vi "Main Worker.vi"(9 "Read Queue Return":refnum<queue>, 10 "Control Queue Return":refnum<queue>, 11 "Network Session Handler in":refnum<class "Network Session Handler.lvclass">) -> ()   [LabVIEW 2019, in "Network Interface.lvlib" / "Network Session Handler.lvclass"]
uses:
  <vilib>/gpm_packages/@cs/Network-Sink/Source/Network Interface/Network Session Handler/Network Session Handler.lvclass
  <vilib>/gpm_packages/@cs/Network-Sink/Source/Network Interface/Message Queue/Message Queue.lvclass
  <vilib>/gpm_packages/@cs/Network-Sink/Source/Network Interface/Network Session Handler/Network Session Handler.lvclass/Network Session Handler.ctl
  <vilib>/gpm_packages/@cs/Network-Sink/Source/Network Interface/Network Session Handler/Session Handler Message Names ENUM.ctl
  <vilib>/gpm_packages/@cs/Network-Sink/Source/Network Interface/Message Queue/Message Queue.lvclass/Message Queue.ctl
  <vilib>/gpm_packages/@cs/Network-Sink/Source/Network Interface/Network Session Handler/Factory Loop Message Names ENUM.ctl
  <vilib>/gpm_packages/@cs/Network-Sink/Source/Network Interface/Connection Handler/Synchronous Write Request.ctl
  <vilib>/gpm_packages/@cs/event-logger/Source/Composed Log/Types/Log Level.ctl
  <vilib>/gpm_packages/@cs/event-logger/Source/Composed Log/LoggerReference/LoggerReference.lvclass/LoggerReference.ctl
  6a8aa042-a92f-476e-a18a-366c18080255.vi
  510cd40e-2ed8-4bdb-87dc-9d54a7f70cf6.vi
  31b7514c-8e2c-4e78-b35a-21c1860db5bd.vi
  c51e2ab3-c1d1-4a5d-a2cc-0a28ab4f9529.vi
  <vilib>/gpm_packages/@cs/Network-Sink/Source/Network Interface/Message Queue/Protected Enqueue.vi
  <vilib>/gpm_packages/@cs/Network-Sink/Source/Network Interface/Message Queue/Dequeue Message.vi
  <vilib>/gpm_packages/@cs/event-logger/Source/Composed Log/LoggerReference/Log.vi
  <vilib>/gpm_packages/@cs/event-logger/Source/Composed Log/LoggerReference/Get Valid Event Time.vi
  <vilib>/gpm_packages/@cs/event-logger/Source/Composed Log/LoggerReference/Remove Stale Logs.vi
  <vilib>/gpm_packages/@cs/Network-Sink/Source/Network Interface/Connection Handler/Connection Handler.lvclass
  <vilib>/gpm_packages/@cs/event-logger/Source/Composed Log/Composed Log.lvlib
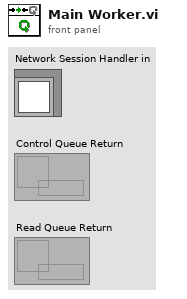
[diagram p1: front panel]
types:
  T1 = typedef "Network Interface.lvlib/Network Session Handler.lvclass/Session Handler Message Names ENUM.ctl" = enum16{"Transmit Message", "Stop", "Handler Shutdown", "Error"}
  T2 = typedef "Network Interface.lvlib/Network Session Handler.lvclass/Factory Loop Message Names ENUM.ctl" = enum16{"Create Connection", "Stop", "Assess Factory State"}
  T3 = typedef "Network Interface.lvlib/Connection Handler.lvclass/Synchronous Write Request.ctl" = cluster{"Data To Write":string, "Return Queue":refnum<queue>}
  T4 = typedef "Composed Log.lvlib/Log Level.ctl" = enum16{"Debug", "Info", "Warning", "Error", "Critical"}
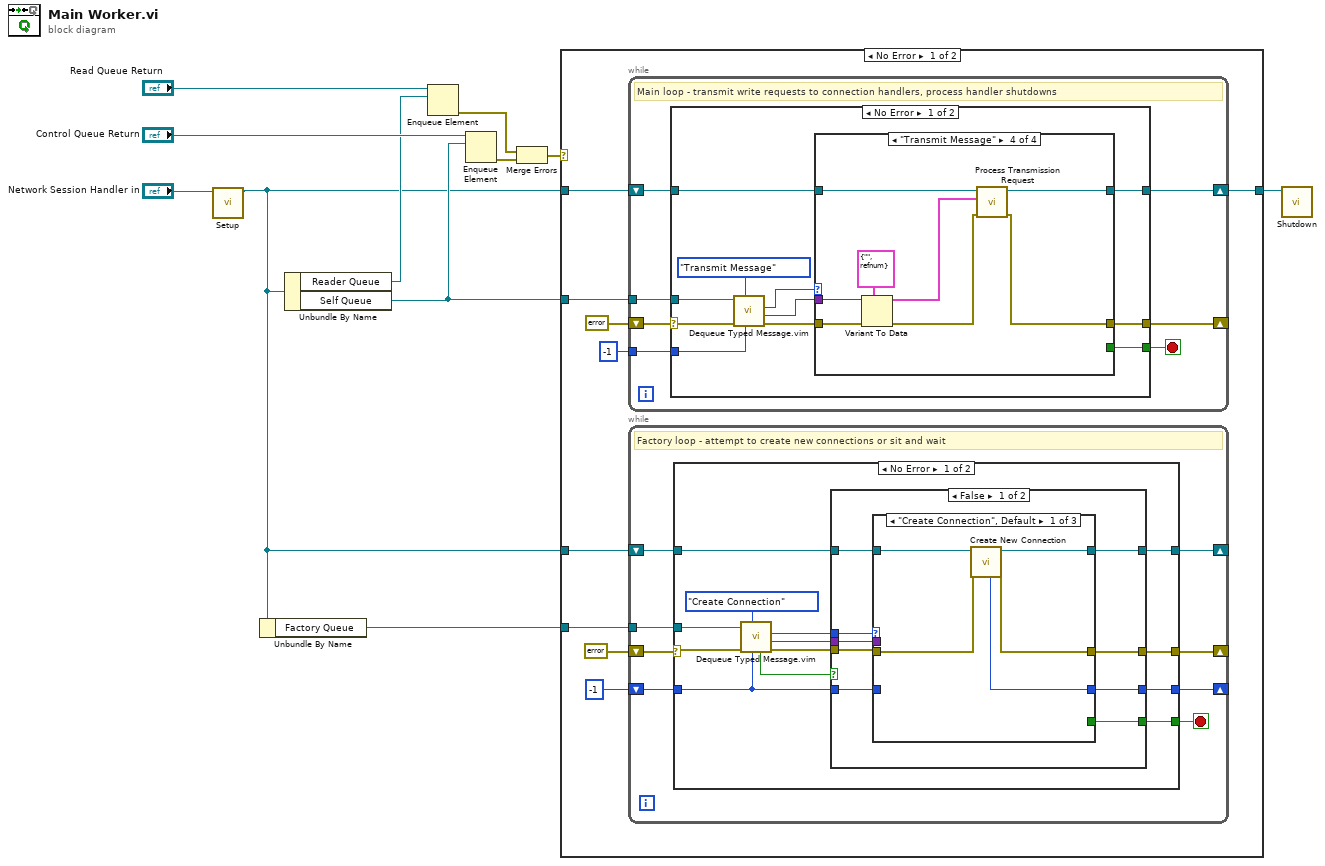
[diagram p0: block diagram]
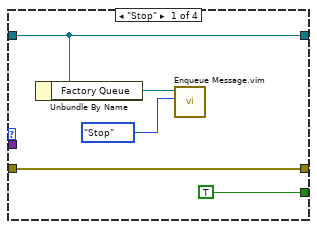
[diagram p2: hidden frame]
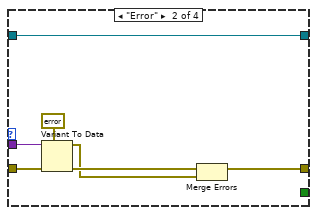
[diagram p3: hidden frame]
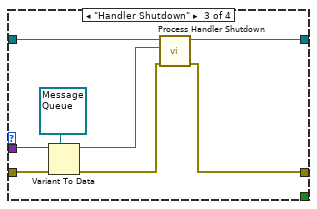
[diagram p4: hidden frame]
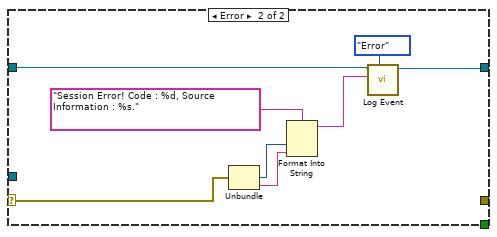
[diagram p5: hidden frame]
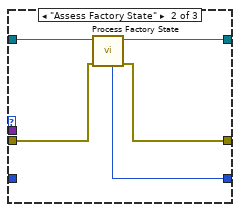
[diagram p6: hidden frame]
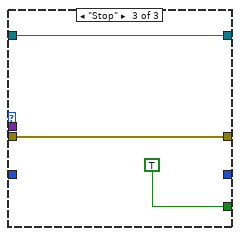
[diagram p7: hidden frame]
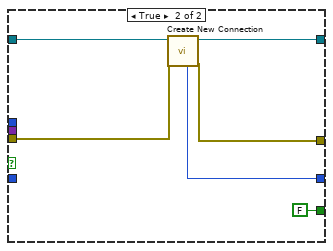
[diagram p8: hidden frame]
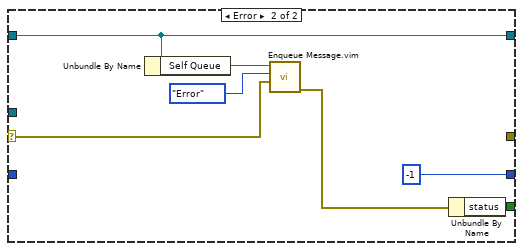
[diagram p9: hidden frame]
diagram:
  n1 = call <vilib>:"Setup.vi"("Network Session Handler in"="Network Session Handler in") -> ("Network Session Handler out"=w1:refnum<class "Network Session Handler.lvclass">)  [unwired: 9 in, 1 out]
  n2 = Unbundle By Name(w1) -> ("Factory Queue"=w11:refnum<class "Message Queue.lvclass">)
  n3 = Unbundle By Name(w1) -> ("Reader Queue"=w6:refnum<queue>, "Self Queue"=w8:refnum<class "Message Queue.lvclass">)
  n4 = Enqueue Element(queue="Read Queue Return", element=w6) -> (error out=w3:errorcluster)  [unwired: 2 in, 2 out]
  n5 = Enqueue Element(queue="Control Queue Return", element=w8) -> (error out=w5:errorcluster)  [unwired: 2 in, 2 out]
  n6 = Merge Errors(w3, w5) -> (w4:errorcluster)
  n7 = case shown="No Error" w4 {
    tunnel: w11 -> [w19 _]
    tunnel: w1 -> [w16 _]
    tunnel: w8 -> [w15 _]
    tunnel: w1 -> [w14 w131]
    tunnel: [w13 w131] -> w2
    frame No Error {
      n8 = while {
        tunnel: w15 -> [w23]
        shift-right: [w27] -> _
        shift-left: errorcluster {"status"=FALSE, "code"=0, "source"=""} ("error out") -> [w24]
        shift-right: [w25] -> w13
        shift-left: w14 -> [w26]
        tunnel: -1 ("Timeout (-1)") -> [w21]
        stop <- w22 stop-if-true
        # "Main loop - transmit write requests to connection handlers, process handler shutdowns"
        n9 = case shown="No Error" w24 {
          selector: w24 -> [w35 w70]
          tunnel: [w38 _] -> w27
          tunnel: w26 -> [w37 w69]
          tunnel: [w36 w68] -> w25
          tunnel: w23 -> [w34 _]
          tunnel: [w29 _] -> w22
          tunnel: w21 -> [w28 _]
          frame No Error {
            n10 = call "Dequeue Typed Message.vim"("Timeout (-1)"=w28, "Type"=Session_Handler_Message_Names_ENUM."Transmit Message", "error in (no error)"=w35, "Message Queue in"=w34) -> ("error out"=w30:errorcluster, "Data"=w31:variant, "Msg"=w32:T1)  [unwired: 3 in, 2 out]
            n11 = case shown="\"Transmit Message\"" w32 {
              tunnel: w31 -> [_ w48 w56 w65]
              tunnel: w30 -> [w43 w50 w58 w66]
              tunnel: [w43 w45 w52 w59] -> w38
              tunnel: w37 -> [w41 w46 w55 w64]
              tunnel: [w41 w46 w54 w63] -> w36
              tunnel: [TRUE _ _ _] -> w29
              frame "Stop" {
                n12 = Unbundle By Name(w41) -> ("Factory Queue"=w40:refnum<class "Message Queue.lvclass">)
                n13 = call "Enqueue Message.vim"("Msg"=Factory_Loop_Message_Names_ENUM."Stop" ("Factory Message Names"), "Message Queue in"=w40) -> ()  [unwired: 8 in, 2 out]
              }
              frame "Error" {
                n14 = Variant To Data(error in=w50, type=errorcluster {"status"=FALSE, "code"=0, "source"=""} ("error out"), Variant=w48) -> (data=w44:errorcluster, error out=w49:errorcluster)
                n15 = Merge Errors(w49, w44) -> (w45:errorcluster)
              }
              frame "Handler Shutdown" {
                n16 = Variant To Data(error in=w58, type=refnum<class "Message Queue.lvclass"> refnum ("Network Sink.lvlib:Message Queue.lvclass"), Variant=w56) -> (data=w51:refnum<class "Message Queue.lvclass">, error out=w53:errorcluster)
                n17 = call <vilib>:"Process Handler Shutdown.vi"("error in (no error)"=w53, "Handler Queue"=w51, "Network Session Handler in"=w55) -> ("error out"=w52:errorcluster, "Network Session Handler out"=w54:refnum<class "Network Session Handler.lvclass">)  [unwired: 7 in]
              }
              frame "Transmit Message" {
                n18 = Variant To Data(error in=w66, type=T3 {"Data To Write"="", "Return Queue"=refnum} ("Write Request"), Variant=w65) -> (data=w61:T3, error out=w60:errorcluster)
                n19 = call <vilib>:"Process Transmission Request.vi"("error in (no error)"=w60, "Write Request"=w61, "Network Session Handler in"=w64) -> ("error out"=w59:errorcluster, "Network Session Handler out"=w63:refnum<class "Network Session Handler.lvclass">)  [unwired: 7 in]
              }
            }
          }
          frame Error {
            n20 = Unbundle(w70) -> ("code"=w73:i32, "source"=w72:string)  [unwired: 1 out]
            n21 = Format Into String(format string="Session Error! Code : %d, Source Information : %s.", w73, w72) -> (resulting string=w67:string)  [unwired: 2 in, 1 out]
            n22 = call <vilib>:"Log Event.vi"("Event Level"=Log_Level."Error", "Event"=w67, "Network Session Handler in"=w69) -> ("Network Session Handler out"=w68:refnum<class "Network Session Handler.lvclass">)  [unwired: 7 in, 1 out]
          }
        }
      }
      n23 = while {
        tunnel: w19 -> [w82]
        shift-right: [w80] -> _
        shift-left: errorcluster {"status"=FALSE, "code"=0, "source"=""} ("error out") -> [w81]
        shift-right: [w77] -> _
        shift-left: -1 ("timeout in ms (-1)") -> [w78]
        shift-right: [w75] -> _
        shift-left: w16 -> [w76]
        stop <- w79 stop-if-true
        # "Factory loop - attempt to create new connections or sit and wait"
        n24 = case shown="No Error" w81 {
          selector: w81 -> [w89 w127]
          tunnel: w82 -> [w90 _]
          tunnel: [w95 _] -> w80
          tunnel: [w94 w130] -> w79
          tunnel: w78 -> [w88 _]
          tunnel: [w93 -1 ("timeout in ms (-1)")] -> w77
          tunnel: w76 -> [w92 w125]
          tunnel: [w91 w125] -> w75
          frame No Error {
            n25 = call "Dequeue Typed Message.vim"("Timeout (-1)"=w88, "Type"=Factory_Loop_Message_Names_ENUM."Create Connection" ("Factory Message Names"), "error in (no error)"=w89, "Message Queue in"=w90) -> ("error out"=w87:errorcluster, "Data"=w85:variant, "Msg"=w86:T2, "Timed Out?"=w84:bool)  [unwired: 3 in, 1 out]
            n26 = case shown="False" w84 {
              tunnel: [w104 w120] -> w95
              tunnel: [w103 FALSE] -> w94
              tunnel: [w102 w119] -> w93
              tunnel: w92 -> [w101 w123]
              tunnel: [w100 w122] -> w91
              tunnel: w88 -> [w99 _]
              tunnel: w87 -> [w98 w121]
              tunnel: w86 -> [w97 _]
              tunnel: w85 -> [w96 _]
              frame False {
                n27 = case shown="\"Create Connection\", Default" w97 {
                  tunnel: [w106 w111 w117] -> w104
                  tunnel: w98 -> [w107 w112 w117]
                  tunnel: [_ _ TRUE] -> w103
                  tunnel: w99 -> [_ _ _]
                  tunnel: [w105 w110 _] -> w102
                  tunnel: w101 -> [w109 w114 w115]
                  tunnel: [w108 w113 w115] -> w100
                  tunnel: w96 -> [_ _ _]
                  frame "Create Connection", Default {
                    n28 = call <vilib>:"Create New Connection.vi"("error in (no error)"=w107, "Network Session Handler in"=w109) -> ("error out"=w106:errorcluster, "Network Session Handler out"=w108:refnum<class "Network Session Handler.lvclass">, "Next Timeout"=w105:i32)  [unwired: 7 in]
                  }
                  frame "Assess Factory State" {
                    n29 = call <vilib>:"Process Factory State.vi"("error in (no error)"=w112, "Network Session Handler in"=w114) -> ("error out"=w111:errorcluster, "Network Session Handler out"=w113:refnum<class "Network Session Handler.lvclass">, "Loop Timeout"=w110:i32)  [unwired: 7 in]
                  }
                  frame "Stop" {
                  }
                }
              }
              frame True {
                n30 = call <vilib>:"Create New Connection.vi"("error in (no error)"=w121, "Network Session Handler in"=w123) -> ("error out"=w120:errorcluster, "Network Session Handler out"=w122:refnum<class "Network Session Handler.lvclass">, "Next Timeout"=w119:i32)  [unwired: 7 in]
              }
            }
          }
          frame Error {
            n31 = Unbundle By Name(w125) -> ("Self Queue"=w124:refnum<class "Message Queue.lvclass">)
            n32 = call "Enqueue Message.vim"("Data"=w127, "Msg"=Session_Handler_Message_Names_ENUM."Error", "Message Queue in"=w124) -> ("error out"=w128:errorcluster)  [unwired: 7 in, 1 out]
            n33 = Unbundle By Name(w128) -> ("status"=w130:bool)
          }
        }
      }
    }
    frame Error {
    }
  }
  n34 = call <vilib>:"Shutdown.vi"("Network Session in"=w2) -> ()  [unwired: 11 in]
